vi "_Axis_Abs.vi"(8 "Error In":errorcluster, 10 "绝对位置":i32, 11 "轴序号":u16) -> (0 "Error Out":errorcluster)   [LabVIEW 2020, in "MT_API.lvlib"]
doc: "MT_API INT32 __stdcall MT_Set_Axis_Position_P_Target_Abs(WORD AObj,INT32 Value);"
uses:
  MT_API.lvlib
  MT_API_64.dll
panel:
  out "函数返回值":i32
  # "将轴移动到绝对位置"
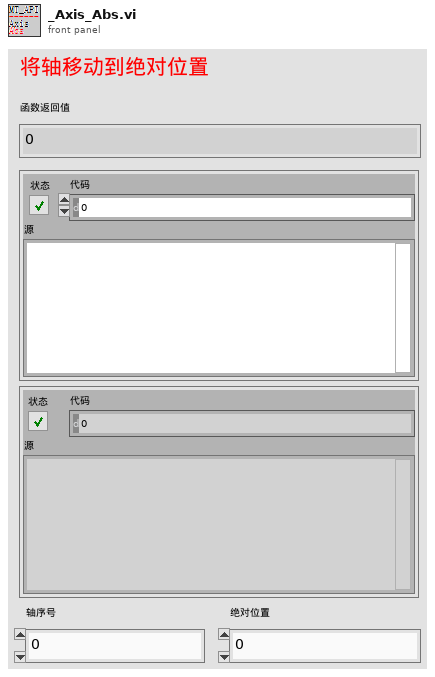
[diagram p1: front panel]
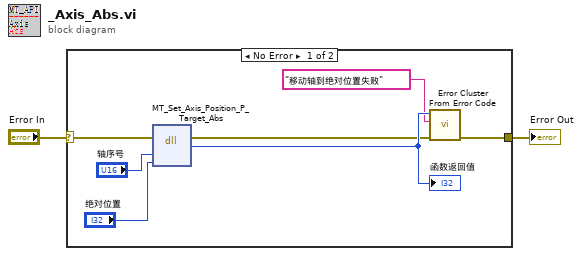
[diagram p0: block diagram]
diagram:
  n1 = case shown="No Error" "Error In" {
    selector: "Error In" -> [w7 w10]
    tunnel: [w3 w10] -> w1
    frame No Error {
      n2 = dll-call lib="D:/Project NJU/lib/MT/MT_API_64.*" fn="MT_Set_Axis_Position_P_Target_Abs"(error in=w7, "AObj"="轴序号", "Value"="绝对位置") -> (error out=w5:errorcluster, "return type"=w6:i32)  [unwired: 4 in, 1 out]
      "函数返回值" <- w6
      n3 = call <vilib>:"Error Cluster From Error Code.vi"("error in (no error)"=w5, "error message (\"\")"="移动轴到绝对位置失败", "error code (0)"=w6) -> ("error out"=w3:errorcluster)  [unwired: 6 in]
    }
    frame Error {
    }
  }
  "Error Out" <- w1
